vi "Read Orient3d.vi"(8 "error in (no error)":errorcluster, 10 "Key":string, 11 "FlexWorktable in":refnum<class "FlexWorktable.lvclass">) -> (0 "error out":errorcluster, 2 "Orient3d out":refnum<class "Orient3d Class.lvclass">, 3 "FlexWorktable out":refnum<class "FlexWorktable.lvclass">)   [LabVIEW 2017, in "FlexWorktable.lvclass"]
uses:
  FlexWorktable.lvclass
  Orient3d Class/Orient3d Class.lvclass
  FlexWorktable.lvclass/FlexWorktable.ctl
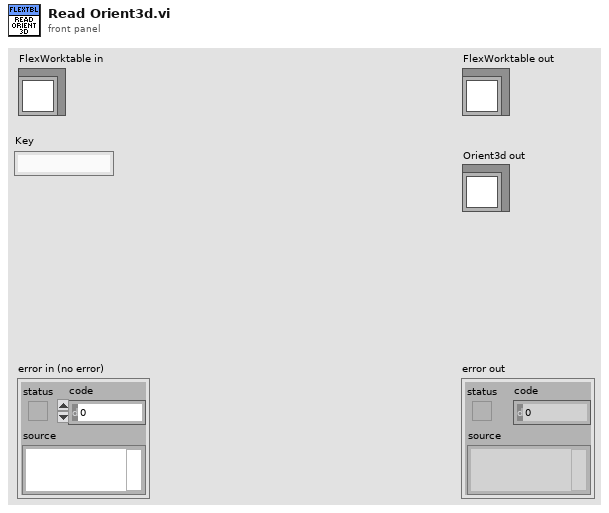
[diagram p1: front panel]
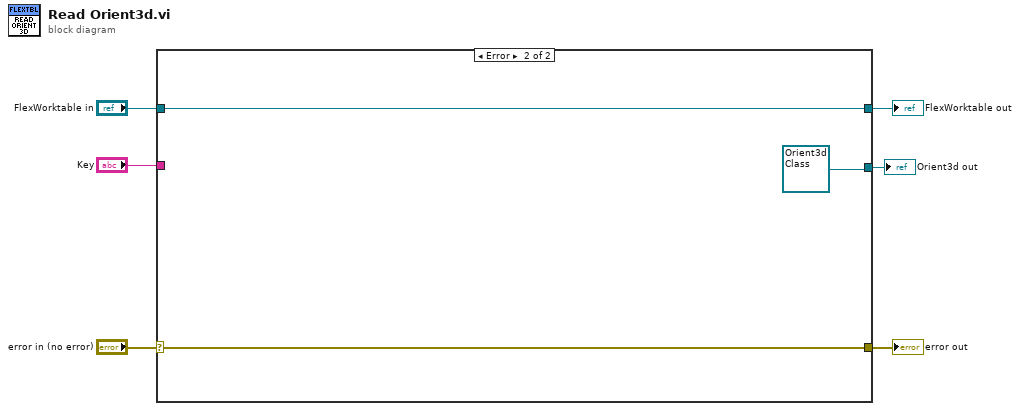
[diagram p0: block diagram]
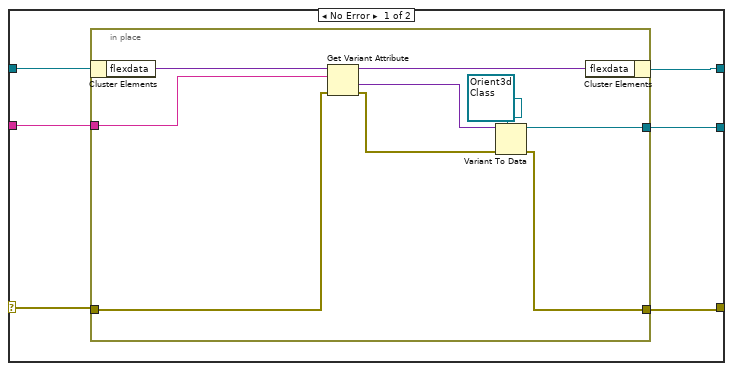
[diagram p2: hidden frame]
diagram:
  n1 = case shown="Error" "error in (no error)" {
    selector: "error in (no error)" -> [w10 w24]
    tunnel: [w7 w24] -> w5
    tunnel: [w8 w23] -> w3
    tunnel: "FlexWorktable in" -> [w12 w23]
    tunnel: "Key" -> [w11 _]
    tunnel: [w9 refnum<class "Orient3d Class.lvclass"> refnum ("Orient3d Class.lvclass")] -> w1
    frame No Error {
      n2 = in-place {
        in-place-border: w11 -> [w19]
        in-place-border: w10 -> [w18]
        in-place-border: [w15] -> w7
        in-place-border: [w14] -> w9
        n3 = in-place-cluster #1(w12) -> ("flexdata"=w21:variant)
        n4 = Get Variant Attribute(Variant=w21, name=w19, error in=w18) -> (duplicate Variant=w20:variant, value=w17:variant, error out=w16:errorcluster)  [unwired: 1 in, 1 out]
        n5 = Variant To Data(error in=w16, type=refnum<class "Orient3d Class.lvclass"> refnum ("Orient3d Class.lvclass"), Variant=w17) -> (data=w14:refnum<class "Orient3d Class.lvclass">, error out=w15:errorcluster)
        n6 = in-place-cluster #1("flexdata"=w20) -> (w8:refnum<class "FlexWorktable.lvclass">)
      }
    }
    frame Error {
    }
  }
  "error out" <- w5
  "FlexWorktable out" <- w3
  "Orient3d out" <- w1
